vi "Thermistor 3.vi"() -> ()   [LabVIEW 2020]
uses:
  <vilib>/ULx/Create Channel.llb/ULx Create Channel (AI-Voltage-Basic).vi
  <vilib>/ULx/Timing.llb/ULx Timing (Sample Clock).vi
  <vilib>/ULx/Read.llb/ULx Read (Analog DBL 1Chan 1Samp).vi
panel:
  in  "Time Target (s)":dbl=1.0
  in  "rate":dbl=1000.0
  in  "samples per channel":i32=1000
  in  "sample mode":i32(ring) items=["FiniteSamples", "ContinuousSamples"]
  in  "physical channels":refnum<k21>
  in  "minimum value":dbl=-5.0
  in  "maximum value":dbl=5.0
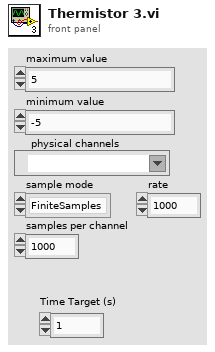
[diagram p1: front panel]
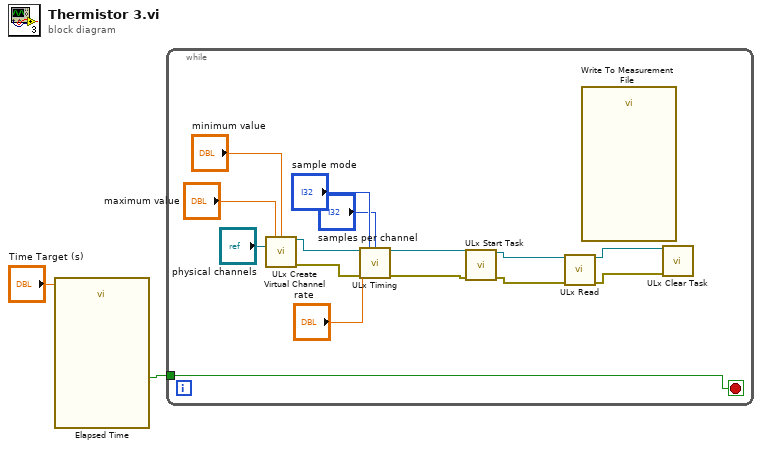
[diagram p0: block diagram]
diagram:
  n1 = call "Elapsed Time"("Time Target (s)"="Time Target (s)") -> ("Time has Elapsed"=w2:bool)  [unwired: 11 in, 7 out]
  n2 = while {
    tunnel: w2 -> [w3]
    stop <- w3 stop-if-true
    n3 = call-poly <vilib>:"ULx Create Virtual Channel.vi"("maximum value"="maximum value", "minimum value"="minimum value", "physical channels"="physical channels") -> ("task out"=w13:refnum<k24>, "error out"=w17:errorcluster)  [unwired: 11 in]
    n4 = call-poly <vilib>:"ULx Timing.vi"("task in"=w13, "sample mode"="sample mode", "samples per channel"="samples per channel", "rate"="rate", "error in"=w17) -> ("task out"=w12:refnum<k24>, "error out"=w16:errorcluster)  [unwired: 9 in]
    n5 = call <vilib>:"ULx Start Task.vi"("task in"=w12, "error in"=w16) -> ("task out"=w11:refnum<k24>, "error out"=w15:errorcluster)  [unwired: 12 in]
    n6 = call-poly <vilib>:"ULx Read.vi"("task in"=w11, "error in"=w15) -> ("task out"=w10:refnum<k24>, "error out"=w14:errorcluster)  [unwired: 11 in, 1 out]
    n7 = call "Write To Measurement File"() -> ()  [unwired: 17 in, 3 out]
    n8 = call <vilib>:"ULx Clear Task.vi"("task in"=w10, "error in"=w14) -> ()  [unwired: 13 in, 1 out]
  }
